vi "Test Format Method Description.vi"(8 "error in (no error)":errorcluster, 11 "Test Result Tree Test in":refnum<class "Test Result Tree Test.lvclass">) -> (0 "error out":errorcluster, 3 "Test Result Tree Test out":refnum<class "Test Result Tree Test.lvclass">)   [LabVIEW 2020, in "Test Result Tree Test.lvclass"]
uses:
  Test Result Tree Test.lvclass
  C:/Program Files (x86)/National Instruments/LabVIEW 2020/vi.lib/Astemes/LUnit/Test Case.lvclass
  Result/Result.ctl
  Result/Status.ctl
  Result/Type.ctl
  Test Result Tree/Test Result Tree V2.lvclass
  C:/Git/astemes-lunit/source/Rewrite Project/Test Tree/Test Tree.lvclass
  LUnit Test Case Tests/LUnit Test Case V2 Test Double/Methods.ctl
  <vilib>/Astemes/LUnit/Test Case.lvclass/Test Case.ctl
  <vilib>/Astemes/LUnit/Palette/Fail.vi
  <vilib>/Astemes/LUnit/Palette/Pass.vi
  <vilib>/Astemes/LUnit/Set Assertion Type.vi
  <vilib>/Astemes/LUnit/Add test result.vi
  <vilib>/Astemes/LUnit/LUnit Record Assertion Result.vi
  <vilib>/Astemes/LUnit/LUnit Aggregate Assertion Results.vi
  <vilib>/Astemes/LUnit/Method Result/LUnit Merge Status.vi
  <vilib>/Astemes/LUnit/LUnit Concatenate result strings.vi
  LUnit Test Case/LUnit Test Case V2.lvclass
  Test Result Tree Test.lvclass/Test Result Tree Test.ctl
  Test Tree/Test Tree.lvclass
  LUnit Test Case Tests/LUnit Test Case V2 Test Double/LUnit Test Case V2 Test Double.lvclass
  <vilib>/Astemes/LUnit/Test Case.lvclass
  Result/Result.lvlib
panel:
  out "Results":T1[](array[typedef])
  out "Description":string
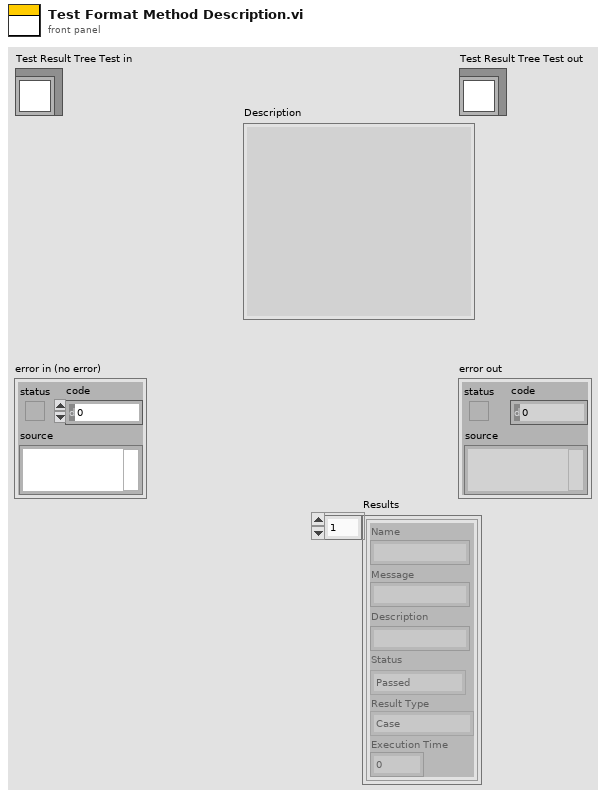
[diagram p1: front panel]
types:
  T1 = typedef "Result.lvlib/Result.ctl" = cluster{"Name":string, "Message":string, "Description":string, "Status":T2, "Result Type":T3, "Execution Time":dbl}
  T2 = typedef "Result.lvlib/Status.ctl" = enum16{"", "Passed", "Failed", "Error", "Skipped", "Setup Error", "Broken", "Teardown Error"}
  T3 = typedef "Result.lvlib/Type.ctl" = enum16{"Method", "Case", "Suite", "Pass", "Fail", "Skip", "Pass if", "Fail if", "Pass if Error", "Fail if Error", "Pass if Equal", "Fail if Equal"}
  T4 = typedef "LUnit Test Case V2 Test Double.lvclass/Methods.ctl" = enum16{"Test Failing Test.vi", "Test Passing Test.vi", "Test Error Test.vi", "Test Skip Test.vi", "Test Passing Pass If Test.vi", "Test Failing Pass If Test.vi", "Test Failing Fail If Test.vi", "Test Passing Fail If Test.vi", "Test Passing Pass If Error Test.vi", "Test Failing Pass If Error Test.vi", "Test Passing Fail If Error Test.vi", "Test Failing Fail If Error Test.vi", "Test Passing Pass If Equal Test.vi", "Test Failing Pass If Equal Test.vi", "Test Failing Fail If Equal Test.vi", "Test Passing Fail If Equal Test.vi"}
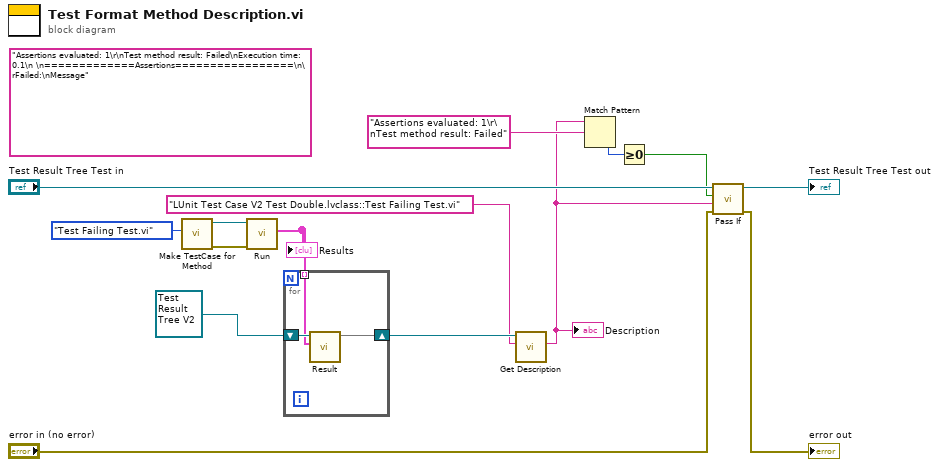
[diagram p0: block diagram]
diagram:
  (unwired) "Assertions evaluated: 1\r\nTest method result: Failed\nExecution time: 0.1\n \n=============Assertions=================\n\rFailed:\nMessage" ("format string")
  n1 = call "Make TestCase for Method.vi"("Test Method"=Methods."Test Failing Test.vi") -> ("error out"=w8:errorcluster, "LUnit Test Case V2 out"=w9:refnum<class "LUnit Test Case V2.lvclass">)  [unwired: 9 in]
  n2 = call-dynamic "Run.vi"("error in (no error)"=w8, "LUnit Test Case V2 in"=w9) -> ("Results"=w5:T1[])  [unwired: 8 in, 1 out]
  "Results" <- w5
  n3 = for {
    shift-right: [w18] -> w12
    shift-left: refnum<class "Test Result Tree V2.lvclass"> refnum ("Test Result Tree V2.lvclass") -> [w17]
    tunnel: w5 -> [w16] mode=indexing
    n4 = call-dynamic "Result.vi"("Result"=w16, "Test Result Tree V2 in"=w17) -> (3:w18)  [unwired: 8 in, 1 out]
  }
  n5 = call "Get Description.vi"("Tag"="LUnit Test Case V2 Test Double.lvclass::Test Failing Test.vi" ("Case"), "Test Tree In"=w12) -> ("Description"=w1:string)  [unwired: 6 in, 3 out]
  "Description" <- w1
  n6 = Match Pattern(string=w1, regular expression="Assertions evaluated: 1\r\nTest method result: Failed" ("format string")) -> (offset past match=w3:i32)  [unwired: 1 in, 3 out]
  n7 = Greater Or Equal To 0?(x=w3) -> (x >= 0?=w2:bool)
  n8 = call <vilib>:"Pass If.vi"("error in (no error)"="error in (no error)", "Message"=w1, "Pass?"=w2, "LUnit Test Case In"="Test Result Tree Test in") -> ("error out"=→"error out":errorcluster, "LUnit Test Case Out"=→"Test Result Tree Test out":refnum<class "Test Result Tree Test.lvclass">)  [unwired: 6 in]
